vi "PM5000_VIF_Alarmas.vi"(8 "error in":errorcluster, 11 "Network Path":string="172.22.26.202") -> (0 "error out":errorcluster, 2 "output cluster":T1, 3 "Network Path out":string="192.168.169.1")   [LabVIEW 2018]
doc: "Lee la tabla de memoria RealTime_VIF_Power del equipo PowerMonitor 5000, ademas filtra y ordena las variables de interez de la tabla de memoria.\n\nLee las siguientes variables de la tabla RealTime_VIF_Power:\n\n*V1_V2_Volts\n*V2_V3_Volts\n*V3_V1_Volts\n*I1_Amps\n*I2_Amps\n*I3_Amps\n*Frequency_Hz\n*Total_kW\n*Total_kVAR\n*Total_kVA\n*Total_True_PF\n*Total_Disp_PF"
uses:
  Controls/VIF_cluster.ctl
  <vilib>/ethernetip/ethernetip.llb/EthernetIP SLC500 Read Float.vi
  <vilib>/ethernetip/ethernetip.lvlib
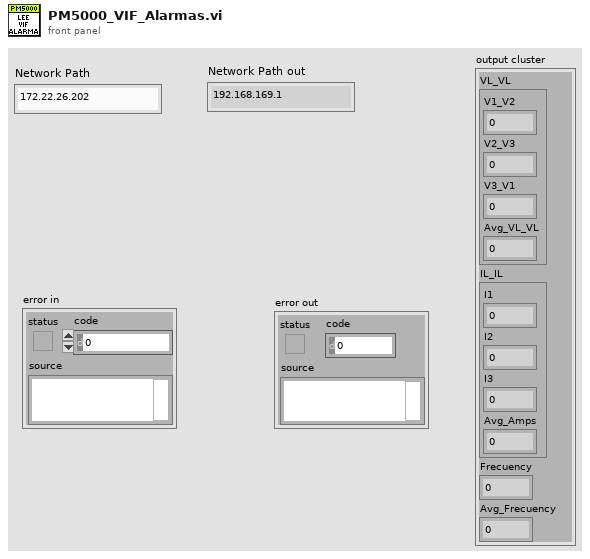
[diagram p1: front panel]
types:
  T1 = typedef "VIF_cluster.ctl" = cluster{"VL_VL":cluster{"V1_V2":sgl, "V2_V3":sgl, "V3_V1":sgl, "Avg_VL_VL":sgl}, "IL_IL":cluster{"I1":sgl, "I2":sgl, "I3":sgl, "Avg_Amps":sgl}, "Frecuency":sgl, "Avg_Frecuency":sgl}
  T2 = cluster{"I1":sgl, "I2":sgl, "I3":sgl, "Avg_Amps":sgl}
  T3 = cluster{"V1_V2":sgl, "V2_V3":sgl, "V3_V1":sgl, "Avg_VL_VL":sgl}
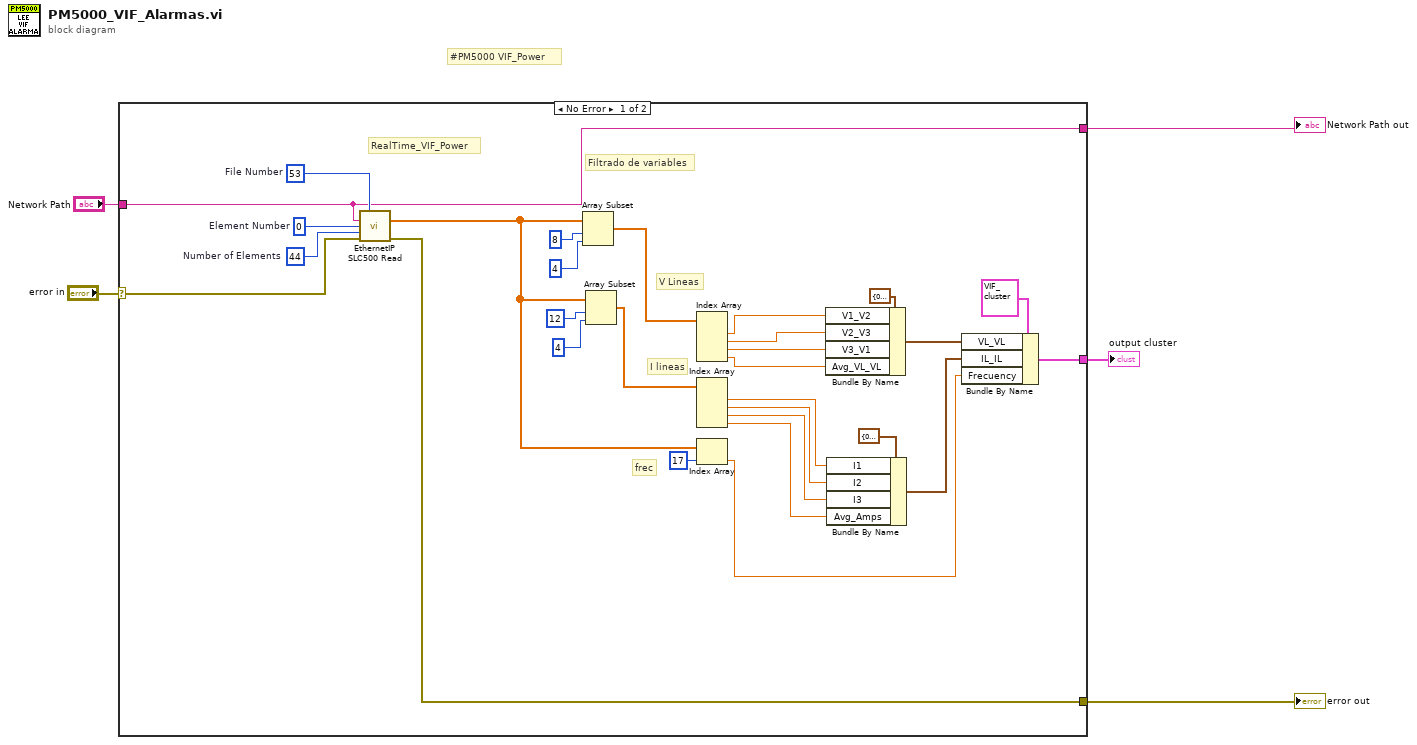
[diagram p0: block diagram]
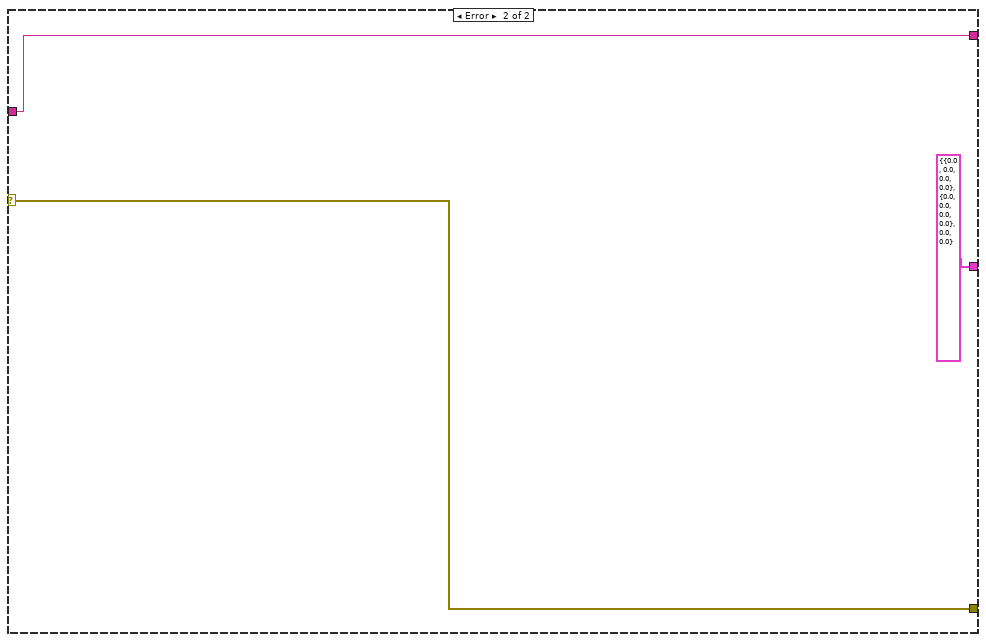
[diagram p2: hidden frame]
diagram:
  # "#PM5000 VIF_Power"
  n1 = case shown="No Error" "error in" {
    selector: "error in" -> [w26 w37]
    tunnel: [w31 w37] -> w5
    tunnel: [w23 w36] -> w3
    tunnel: "Network Path" -> [w23 w36]
    tunnel: [w6 T1 {"VL_VL"={"V1_V2"=0.0, "V2_V3"=0.0, "V3_V1"=0.0, "Avg_VL_VL"=0.0}, "IL_IL"={"I1"=0.0, "I2"=0.0, "I3"=0.0, "Avg_Amps"=0.0}, "Frecuency"=0.0, "Avg_Frecuency"=0.0} ("VIF_cluster")] -> w1
    frame No Error {
      w32 = u32 44  # Number of Elements
      w34 = u16 53  # File Number
      w33 = u16 0  # Element Number
      # "frec"
      # "I lineas"
      # "V Lineas"
      # "Filtrado de variables"
      # "RealTime_VIF_Power"
      n2 = call-poly <vilib>:"EthernetIP SLC500 Read.vi"("File Number"=w34, "Network Path"=w23, "Element Number"=w33, "Number of Elements"=w32, "error in"=w26) -> ("Data"=w21:sgl[], "error out"=w31:errorcluster)  [unwired: 8 in, 1 out]
      n3 = Array Subset(array=w21, index=8, length=4) -> (w25:sgl[])
      n4 = Array Subset(array=w21, index=12, length=4) -> (w24:sgl[])
      n5 = Index Array(array=w25) -> (element #1=w15:sgl, element #2=w14:sgl, element #3=w13:sgl, element #4=w12:sgl)  [unwired: 4 in]
      n6 = Index Array(array=w24) -> (element #1=w11:sgl, element #2=w10:sgl, element #3=w9:sgl, element #4=w8:sgl)  [unwired: 4 in]
      n7 = Index Array(array=w21, index=17) -> (element=w7:sgl)
      n8 = Bundle By Name(cluster=T3 {"V1_V2"=0.0, "V2_V3"=0.0, "V3_V1"=0.0, "Avg_VL_VL"=0.0} ("VL_VL"), "V1_V2"=w15, "V2_V3"=w14, "V3_V1"=w13, "Avg_VL_VL"=w12) -> (w19:T3)
      n9 = Bundle By Name(cluster=T2 {"I1"=0.0, "I2"=0.0, "I3"=0.0, "Avg_Amps"=0.0} ("IL_IL"), "I1"=w11, "I2"=w10, "I3"=w9, "Avg_Amps"=w8) -> (w17:T2)
      n10 = Bundle By Name(cluster=T1 {"VL_VL"={"V1_V2"=0.0, "V2_V3"=0.0, "V3_V1"=0.0, "Avg_VL_VL"=0.0}, "IL_IL"={"I1"=0.0, "I2"=0.0, "I3"=0.0, "Avg_Amps"=0.0}, "Frecuency"=0.0, "Avg_Frecuency"=0.0} ("VIF_cluster"), "VL_VL"=w19, "IL_IL"=w17, "Frecuency"=w7) -> (w6:T1)
    }
    frame Error {
    }
  }
  "error out" <- w5
  "Network Path out" <- w3
  "output cluster" <- w1
